vi "get_serial_string.vi"(4 "Error in":errorcluster, 6 "Semaphore in":T1, 7 "VISA resource name in":refnum<visa-resource-name>) -> (0 "Error out":errorcluster, 1 "Serial response":string, 2 "Semaphore out":T1, 3 "VISA resource name out":refnum<visa-resource-name>)   [LabVIEW 2010]
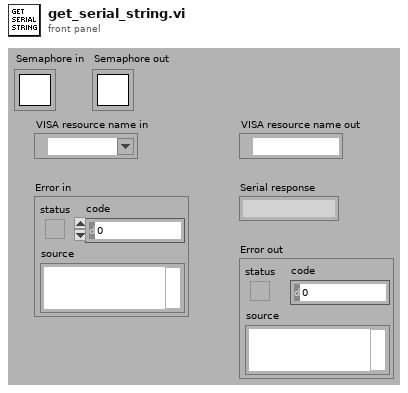
[diagram p1: front panel]
types:
  T1 = typedef "Semaphore RefNum" = refnum<k1>
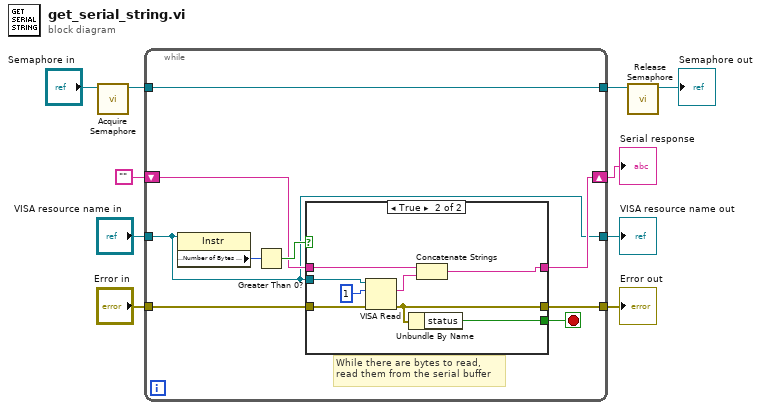
[diagram p0: block diagram]
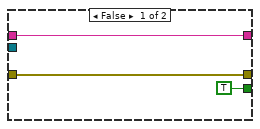
[diagram p2: hidden frame]
diagram:
  n1 = call <vilib>:"Acquire Semaphore.vi"("semaphore"="Semaphore in") -> ("semaphore out"=w4:T1)  [unwired: 4 in, 2 out]
  n2 = while {
    tunnel: "VISA resource name in" -> [w12]
    shift-right: [w16] -> w10
    shift-left: "" -> [w17]
    tunnel: "Error in" -> [w15]
    tunnel: [w14] -> w8
    tunnel: [w12] -> w9
    tunnel: w4 -> [w11]
    tunnel: [w11] -> w2
    stop <- w13 stop-if-true
    # "While there are bytes to read,\nread them from the serial buffer"
    n3 = property class="Instr"(reference=w12) -> ("Serial Settings:Number of Bytes at Serial Port"=w19:u32)  [unwired: 1 in, 2 out]
    n4 = Greater Than 0?(x=w19) -> (x > 0?=w18:bool)
    n5 = case shown="True" w18 {
      tunnel: w17 -> [w20 w30]
      tunnel: [w20 w29] -> w16
      tunnel: w12 -> [_ w26]
      tunnel: w15 -> [w22 w25]
      tunnel: [w22 w24] -> w14
      tunnel: [TRUE w23] -> w13
      frame False {
      }
      frame True {
        n6 = VISA Read(VISA resource name=w26, byte count=u32 1, error in (no error)=w25) -> (read buffer=w28:string, error out=w24:errorcluster)  [unwired: 2 out]
        n7 = Unbundle By Name(w24) -> ("status"=w23:bool)
        n8 = Concatenate Strings(w30, w28) -> (w29:string)
      }
    }
  }
  "Serial response" <- w10
  "VISA resource name out" <- w9
  "Error out" <- w8
  n9 = call <vilib>:"Release Semaphore.vi"("semaphore"=w2) -> ("semaphore out"=→"Semaphore out":T1)  [unwired: 5 in, 1 out]
